vi "chaos crest push time.vi"(9 "min_time":u32, 10 "max_time":u32, 11 "h":u32) -> (1 "min_time out":u32, 2 "max_time out":u32, 3 "h out":u32, 5 "function return":sgl)   [LabVIEW 2014, in "libcommon-crest.lvlib"]
doc: "float chaos_crest_push_time(chaos_crest_handle_t h,uint32_t*max_time,uint32_t*min_time);"
uses:
  libcommon-crest.lvlib
  chaos-i686-dynamic-release/lib/libcommon-crest.so
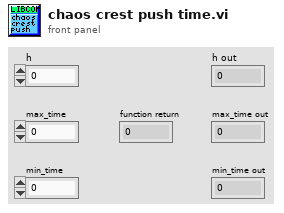
[diagram p1: front panel]
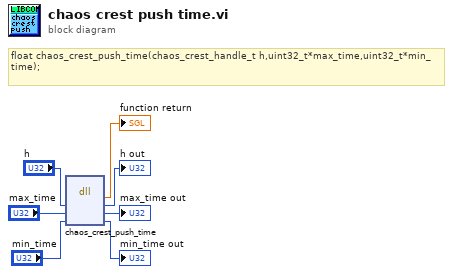
[diagram p0: block diagram]
diagram:
  # "float chaos_crest_push_time(chaos_crest_handle_t h,uint32_t*max_time,uint32_t*min_time);"
  n1 = dll-call lib="home/chaos/chaos_bundle/chaos-i686-dynamic-release/lib/libcommon-crest.*" fn="chaos_crest_push_time"("h"="h", "max_time"="max_time", "min_time"="min_time") -> (→"function return":sgl, "h"=→"h out":u32, "max_time"=→"max_time out":u32, "min_time"=→"min_time out":u32)  [unwired: 3 in, 2 out]
